vi "ShowMouseRoi.vi"(6 "Refnum Image In":T1, 7 "Show mouse selection":bool, 10 "File Path for Mouse Mask":path, 11 "Refnum MouseROI":T1) -> (3 "Refnum Image out":T1)   [LabVIEW 2013]
uses:
  <vilib>/vision/Image Controls.llb/IMAQ Image.ctl
  <vilib>/vision/NI_Vision_Development_Module.lvlib
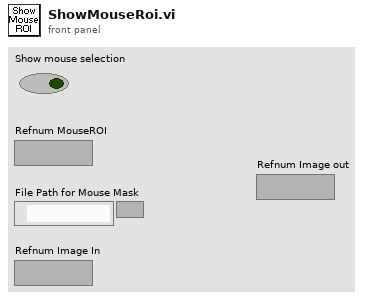
[diagram p1: front panel]
types:
  T1 = typedef "IMAQ Image.ctl" = refnum<image>
  T2 = typedef "ROI Descriptor" = cluster{"Global Rectangle":i32[], "Contours":cluster{"ID":enum32{"External", "Internal"}, "Type":u32, "Coordinates":i32[]}[]}
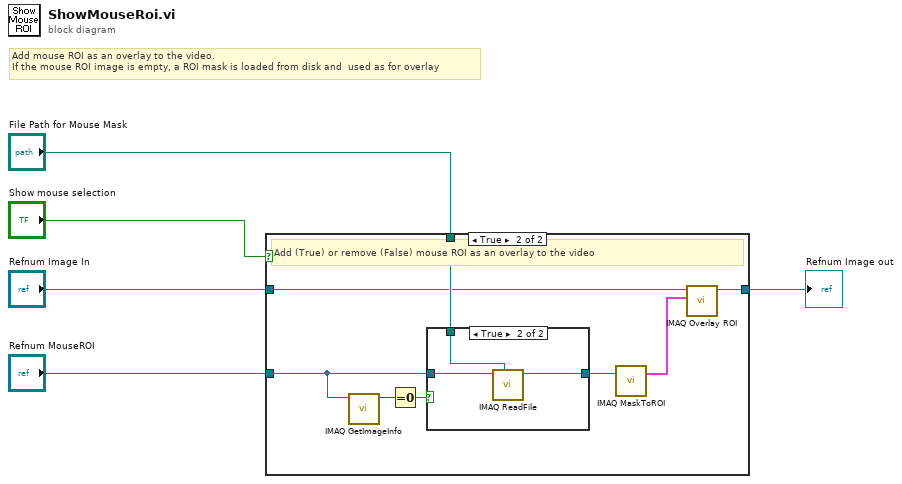
[diagram p0: block diagram]
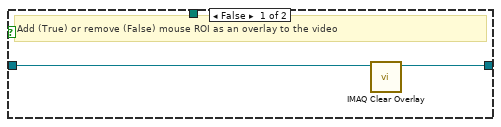
[diagram p2: hidden frame]
diagram:
  # "Add mouse ROI as an overlay to the video.\nIf the mouse ROI image is empty, a ROI mask is loaded from disk and  used as for overlay"
  n1 = case shown="True" "Show mouse selection" {
    tunnel: "Refnum MouseROI" -> [_ w12]
    tunnel: "Refnum Image In" -> [w7 w8]
    tunnel: [w6 w14] -> w3
    tunnel: "File Path for Mouse Mask" -> [_ w13]
    frame False {
      # "Add (True) or remove (False) mouse ROI as an overlay to the video"
      n2 = call "IMAQ Clear Overlay"("Image"=w7) -> ("Image Out"=w6:T1)  [unwired: 9 in, 1 out]
    }
    frame True {
      # "Add (True) or remove (False) mouse ROI as an overlay to the video"
      n3 = call "IMAQ GetImageInfo"("Image"=w12) -> ("X Resolution"=w9:i32)  [unwired: 3 in, 7 out]
      n4 = Equal To 0?(x=w9) -> (x = 0?=w10:bool)
      n5 = case shown="True" w10 {
        tunnel: w13 -> [_ w19]
        tunnel: w12 -> [w16 w18]
        tunnel: [w16 w17] -> w11
        frame False {
        }
        frame True {
          n6 = call "IMAQ ReadFile"("File Path"=w19, "Image"=w18) -> ("Image Out"=w17:T1)  [unwired: 5 in, 4 out]
        }
      }
      n7 = call "IMAQ MaskToROI"("Image"=w11) -> ("ROI Descriptor"=w15:T2)  [unwired: 6 in, 2 out]
      n8 = call "IMAQ Overlay ROI"("ROI Descriptor"=w15, "Image"=w8) -> ("Image Out"=w14:T1)  [unwired: 8 in, 1 out]
    }
  }
  "Refnum Image out" <- w3
